vi "niRFUtil RFHS CONV 1 Ohm Watt to dBm (real wfm).vi"(7 "Real Waveform (W)":T1 {"y" min=0 max=127 format="%.2f"; "dx" format="%^.2e"; "x0" format="%^.2e"}, 11 "error in (no error)":errorcluster) -> (8 "Real Waveform (dBm)":T1 {"y" min=0 max=127 format="%.2f"; "dx" format="%^.2e"; "x0" format="%^.2e"}, 15 "error out":errorcluster)   [LabVIEW 2015, in "niRFUtil.lvlib"]
uses:
  niRFUtil.lvlib
  Includes/niRFUtil INC Real Waveform.ctl
  Includes/niRFUtil INC Real Array.ctl
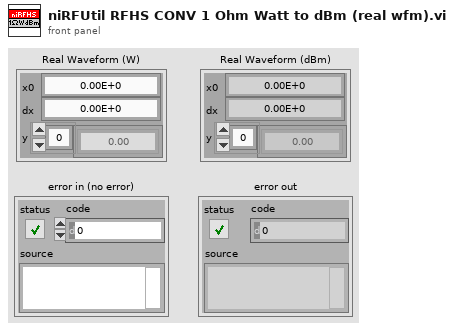
[diagram p1: front panel]
types:
  T1 = typedef "niRFUtil.lvlib/niRFUtil INC Real Waveform.ctl" = cluster{"x0":dbl, "dx":dbl, "y":T2}
  T2 = typedef "niRFUtil.lvlib/niRFUtil INC Real Array.ctl" = sgl[]
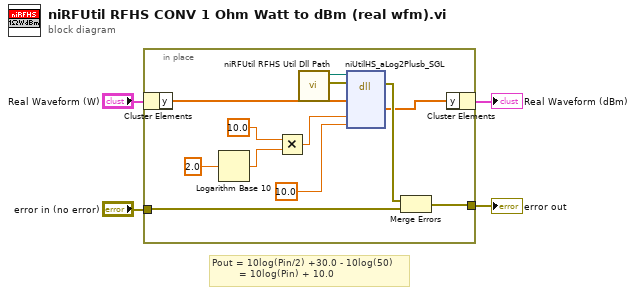
[diagram p0: block diagram]
diagram:
  # "Pout = 10log(Pin/2) +30.0 - 10log(50)\n         = 10log(Pin) + 10.0"
  n1 = in-place {
    in-place-border: "error in (no error)" -> [w6]
    in-place-border: [w5] -> w1
    n2 = in-place-cluster #1("Real Waveform (W)") -> ("y"=w8:T2)
    n3 = Logarithm Base 10(1:sgl 2.0 ("x")) -> (0:w14:sgl)
    n4 = Multiply(x=sgl 10.0, y=w14) -> (x*y=w13:sgl)
    n5 = call "niRFUtil RFHS Util Dll Path.vi"() -> ("error out"=w10:errorcluster, "Path"=w11:path)  [unwired: 7 in, 3 out]
    n6 = dll-call lib="M:/RfProtocols/RFmx/DLLs/niRFHS/trunk/2.1/dist/win32U/niRFHS_avx.dll" fn="niUtilHS_aLog2Plusb_SGL" label="a*log2(x)+b"(path in=w11, error in=w10, "iBuf"=w8, "a"=w13, "b"=sgl 10.0) -> (error out=w9:errorcluster, "oBuf"=w7:sgl[])  [unwired: 6 in, 1 out]
    n7 = Merge Errors(w9, w6) -> (w5:errorcluster)
    n8 = in-place-cluster #1("y"=w7) -> (→"Real Waveform (dBm)":T1)
  }
  "error out" <- w1
